vi "Begin.vi"() -> (0 "error out":errorcluster)   [LabVIEW 2013]
doc: "Called before other user functions, this VI is expected to open initial I/O refnums, load in file data, and do all program initialization. Notice that the <B>error out</B> terminal is simply used for data flow. Wiring it to other structures or subVIs ensures that this VI runs first."
uses:
  <vilib>/Rock Robotics/WPI/Joystick/WPI_JoystickDeviceEnum.ctl
  RefnameEnum.ctl
  RollerAction.ctl
  DoubleSolenoidAction.ctl
  CollectorAction.ctl
  <vilib>/Rock Robotics/SystemInterfaces/Typedef/FPGA_TypedefSolenoidModule.ctl
  <vilib>/Rock Robotics/WPI/Solenoid/WPI_SolenoidChannel.ctl
  <vilib>/Rock Robotics/SystemInterfaces/DIO/FPGA_DIOPWMChannel.ctl
  <vilib>/Rock Robotics/SystemInterfaces/Typedef/FPGA_TypedefDigitalModule.ctl
  <vilib>/Rock Robotics/SystemInterfaces/DIO/FPGA_DIOChannel.ctl
  <vilib>/Rock Robotics/SystemInterfaces/DIO/FPGA_DIORelayChannel.ctl
  <vilib>/Rock Robotics/WPI/Relay/WPI_RelayDirection.ctl
  <vilib>/Rock Robotics/WPI/Solenoid/WPI_SolenoidOpenSingle.vi
  <vilib>/Rock Robotics/WPI/MotorControl/WPI_MotorControlOpen Talon.vi
  <vilib>/Rock Robotics/WPI/Compressor/WPI_CompressorGetSetRefNum.vi
panel:
  # "SET AS DEFAULT"
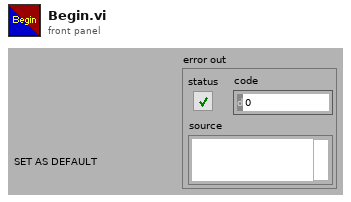
[diagram p1: front panel]
types:
  T1 = typedef "FPGA_DIOChannel.ctl" = enum8{"DIO 1", "DIO 2", "DIO 3", "DIO 4", "DIO 5", "DIO 6", "DIO 7", "DIO 8", "DIO 9", "DIO 10", "DIO 11", "DIO 12", "DIO 13", "DIO 14", "Invalid"}
  T2 = typedef "WPI_RelayDirection.ctl" = enum16{"Both directions", "Forward only", "Reverse only"}
  T3 = typedef "FPGA_DIORelayChannel.ctl" = enum8{"Relay 1", "Relay 2", "Relay 3", "Relay 4", "Relay 5", "Relay 6", "Relay 7", "Relay 8", "Invalid"}
  T4 = typedef "FPGA_TypedefDigitalModule.ctl" = enum16{"Digital Module 1", "Digital Module 2"}
  T5 = typedef "FPGA_DIOPWMChannel.ctl" = enum8{"PWM 1", "PWM 2", "PWM 3", "PWM 4", "PWM 5", "PWM 6", "PWM 7", "PWM 8", "PWM 9", "PWM 10", "Invalid"}
  T6 = typedef "WPI_SolenoidChannel.ctl" = enum8{"Solenoid 1", "Solenoid 2", "Solenoid 3", "Solenoid 4", "Solenoid 5", "Solenoid 6", "Solenoid 7", "Solenoid 8", "Invalid"}
  T7 = typedef "FPGA_TypedefSolenoidModule.ctl" = enum16{"Solenoid Module 1", "Solenoid Module 2"}
  T8 = typedef "CollectorAction.ctl" = enum16{"Init", "Raise", "Lower", "Stop", "GetStatus"}
  T9 = typedef "DoubleSolenoidAction.ctl" = enum16{"Init", "Middle", "In", "Out"}
  T10 = typedef "RefnameEnum.ctl" = enum16{"TankDrive", "Controller1", "Controller2", "SonicShifter", "Compressor"}
  T11 = typedef "RollerAction.ctl" = enum16{"Init", "Off", "Forward", "Reverse"}
  T12 = typedef "WPI_JoystickDeviceEnum.ctl" = enum16{"USB 1", "USB 2", "USB 3", "USB 4", "Kinect 1", "Kinect 2"}
  T13 = typedef "WPI_JoystickDevRef.ctl" = cluster{"Device":T12}
  T14 = typedef "WPI_MotorControlDeviceRef.ctl" = cluster{"DeviceStatus":errorcluster, "Type":enum16{"PWM", "CAN"}, "PWM":cluster{"Digital Module":T4, "PWM Channel":T5, "DeadBand":T15}, "CAN":cluster{"Device Number":u8, "Control Mode":T16, "Semaphore":T17, "Max Vout":dbl}, "Invert":bool, "TransformRef":T18, "InvTransformRef":T18}
  T15 = typedef "WPI_PWMDeadband.ctl" = cluster{"Name":string, "maxPositivePwm":i32, "minPositivePwm":i32, "centerPwm":i32, "maxNegativePwm":i32, "minNegativePwm":i32, "angularRange":u16}
  T16 = typedef "WPI_CANJaguar_ControlMode.ctl" = enum8{"Percent VBus", "Current", "Speed", "Position", "Voltage"}
  T17 = typedef "Semaphore RefNum" = refnum<k1>
  T18 = typedef "WPI_PWMTransform_ConPane.ctl" = refnum<vi>
  T19 = typedef "WPI_DigitalInputDevRef.ctl" = cluster{"DevStatus":errorcluster, "DIO Channel":T1, "Digital Module":T4}
  T20 = typedef "WPI_CompressorDevRef.ctl" = cluster{"DevStatus":errorcluster, "DigitalInputDevRef":T19, "RelayDevRef":T21}
  T21 = typedef "WPI_RelayDevRef.ctl" = cluster{"DevStatus":errorcluster, "Relay Channel":T3, "Digital Module":T4, "Relay Direction":T2}
  T22 = typedef "WPI_SolenoidDevRef.ctl" = cluster{"DevStatus":errorcluster, "Solenoid Module":T7, "Forward Solenoid Channel":T6, "Reverse Solenoid Channel":T6}
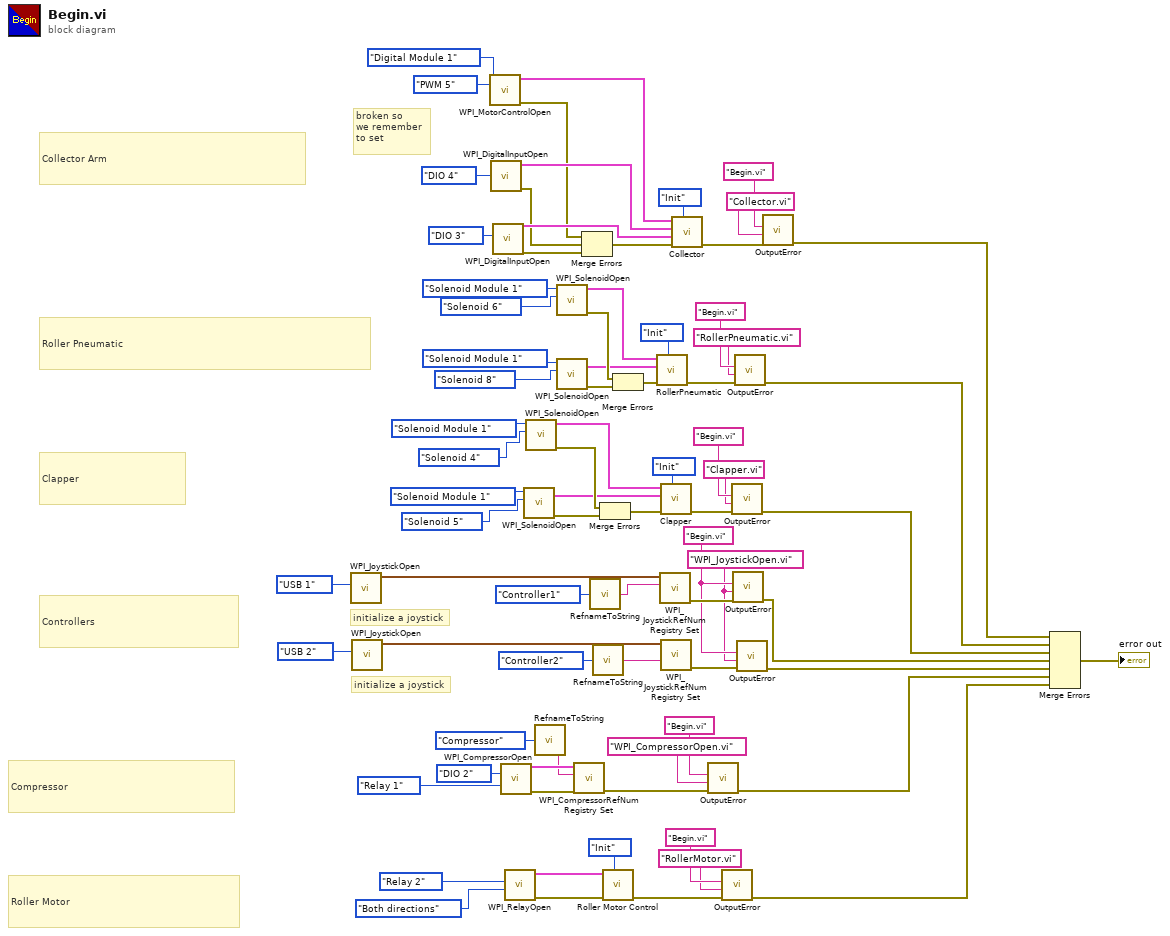
[diagram p0: block diagram]
diagram:
  w70 = "WPI_JoystickOpen.vi" ("Causing VI")
  w71 = "Begin.vi" ("Calling VI")
  # "broken so\nwe remember\nto set"
  # "Collector Arm"
  # "Roller Pneumatic"
  # "Clapper"
  # "Compressor"
  # "Roller Motor"
  # "Controllers"
  # "initialize a joystick"
  # "initialize a joystick"
  n1 = call <vilib>:"WPI_JoystickOpen.vi"("JoystickDevice"=WPI_JoystickDeviceEnum."USB 1") -> ("JoystickDevRef"=w77:T13)  [unwired: 10 in]
  n2 = call <vilib>:"WPI_JoystickOpen.vi"("JoystickDevice"=WPI_JoystickDeviceEnum."USB 2") -> ("JoystickDevRef"=w74:T13)  [unwired: 10 in]
  n3 = call-poly <vilib>:"WPI_MotorControlOpen.vi"("PWM Channel"=FPGA_DIOPWMChannel."PWM 5", "Digital Module (Module 1)"=FPGA_TypedefDigitalModule."Digital Module 1") -> ("error out"=w30:errorcluster, "MotorControlDeviceRef"=w36:T14)  [unwired: 8 in]
  n4 = call <vilib>:"WPI_DigitalInputOpen.vi"("DIO Channel"=FPGA_DIOChannel."DIO 4") -> ("error out"=w31:errorcluster, "DigitalInputDevRef"=w35:T19)  [unwired: 9 in]
  n5 = call <vilib>:"WPI_DigitalInputOpen.vi"("DIO Channel"=FPGA_DIOChannel."DIO 3") -> ("error out"=w32:errorcluster, "DigitalInputDevRef"=w34:T19)  [unwired: 9 in]
  n6 = call <vilib>:"WPI_CompressorOpen.vi"("Pressure Switch DIO Channel"=FPGA_DIOChannel."DIO 2", "Relay Channel"=FPGA_DIORelayChannel."Relay 1") -> ("CompressorDevRef"=w60:T20, "error out"=w59:errorcluster)  [unwired: 3 in, 9 out]
  n7 = call <vilib>:"WPI_RelayOpen.vi"("Relay Direction"=WPI_RelayDirection."Both directions", "Relay Channel"=FPGA_DIORelayChannel."Relay 2") -> ("error out"=w65:errorcluster, "RelayDevRef"=w63:T21)  [unwired: 8 in]
  n8 = call-poly <vilib>:"WPI_SolenoidOpen.vi"("Solenoid Channel"=WPI_SolenoidChannel."Solenoid 5", "Solenoid Module (Module 1)"=FPGA_TypedefSolenoidModule."Solenoid Module 1") -> ("error out"=w23:errorcluster, "SolenoidDevRef"=w22:T22)  [unwired: 8 in]
  n9 = call-poly <vilib>:"WPI_SolenoidOpen.vi"("Solenoid Channel"=WPI_SolenoidChannel."Solenoid 4", "Solenoid Module (Module 1)"=FPGA_TypedefSolenoidModule."Solenoid Module 1") -> ("error out"=w52:errorcluster, "SolenoidDevRef"=w51:T22)  [unwired: 8 in]
  n10 = call "RefnameToString.vi"("Enum"=RefnameEnum."Compressor") -> ("Refname"=w56:string)
  n11 = call-poly <vilib>:"WPI_SolenoidOpen.vi"("Solenoid Channel"=WPI_SolenoidChannel."Solenoid 6", "Solenoid Module (Module 1)"=FPGA_TypedefSolenoidModule."Solenoid Module 1") -> ("error out"=w42:errorcluster, "SolenoidDevRef"=w43:T22)  [unwired: 8 in]
  n12 = call-poly <vilib>:"WPI_SolenoidOpen.vi"("Solenoid Channel"=WPI_SolenoidChannel."Solenoid 8", "Solenoid Module (Module 1)"=FPGA_TypedefSolenoidModule."Solenoid Module 1") -> ("error out"=w18:errorcluster, "SolenoidDevRef"=w17:T22)  [unwired: 8 in]
  n13 = call <vilib>:"WPI_CompressorRefNum Registry Set.vi"("error in (no error)"=w59, "refnum name"=w56, "CompressorDevRef"=w60) -> ("error out"=w58:errorcluster)  [unwired: 7 in, 1 out]
  n14 = Merge Errors(w30, w31, w32) -> (w33:errorcluster)
  n15 = call "RefnameToString.vi"("Enum"=RefnameEnum."Controller1") -> ("Refname"=w68:string)
  n16 = call "RefnameToString.vi"("Enum"=RefnameEnum."Controller2") -> ("Refname"=w66:string)
  n17 = Merge Errors(w52, w23) -> (w24:errorcluster)
  n18 = call "Roller Motor Control.vi"("Action"=RollerAction."Init" ("RollerState"), "Error in"=w65, "RelayDevRef"=w63) -> ("Error out"=w64:errorcluster)  [unwired: 8 in]
  n19 = Merge Errors(w42, w18) -> (w19:errorcluster)
  n20 = call "RollerPneumatic.vi"("State"=DoubleSolenoidAction."Init", "Error in"=w19, "Plugged"=w17, "Open"=w43) -> ("Error out"=w46:errorcluster)  [unwired: 7 in]
  n21 = call <vilib>:"WPI_JoystickRefNum Registry Set.vi"("refnum name"=w68, "JoystickDevRef"=w77) -> ("error out"=w72:errorcluster)  [unwired: 8 in, 1 out]
  n22 = call "Clapper.vi"("State"=DoubleSolenoidAction."Init", "Error in"=w24, "Plugged"=w22, "Open"=w51) -> ("Error out"=w50:errorcluster)  [unwired: 7 in]
  n23 = call <vilib>:"WPI_JoystickRefNum Registry Set.vi"("refnum name"=w66, "JoystickDevRef"=w74) -> ("error out"=w73:errorcluster)  [unwired: 8 in, 1 out]
  n24 = call "Collector.vi"("Action"=CollectorAction."Init", "Error in"=w33, "BottomLS"=w34, "TopLS"=w35, "Motor"=w36) -> ("Error out"=w38:errorcluster)  [unwired: 4 in, 2 out]
  n25 = call "OutputError.vi"("error in (no error)"=w58, "Causing VI"="WPI_CompressorOpen.vi", "Calling VI"="Begin.vi") -> ("error out"=w2:errorcluster)  [unwired: 8 in]
  n26 = call "OutputError.vi"("error in (no error)"=w64, "Causing VI"="RollerMotor.vi", "Calling VI"="Begin.vi") -> ("error out"=w1:errorcluster)  [unwired: 8 in]
  n27 = call "OutputError.vi"("error in (no error)"=w50, "Causing VI"="Clapper.vi", "Calling VI"="Begin.vi") -> ("error out"=w27:errorcluster)  [unwired: 8 in]
  n28 = call "OutputError.vi"("error in (no error)"=w72, "Causing VI"=w70, "Calling VI"=w71) -> ("error out"=w26:errorcluster)  [unwired: 8 in]
  n29 = call "OutputError.vi"("error in (no error)"=w46, "Causing VI"="RollerPneumatic.vi", "Calling VI"="Begin.vi") -> ("error out"=w28:errorcluster)  [unwired: 8 in]
  n30 = call "OutputError.vi"("error in (no error)"=w73, "Causing VI"=w70, "Calling VI"=w71) -> ("error out"=w25:errorcluster)  [unwired: 8 in]
  n31 = call "OutputError.vi"("error in (no error)"=w38, "Causing VI"="Collector.vi", "Calling VI"="Begin.vi") -> ("error out"=w29:errorcluster)  [unwired: 8 in]
  n32 = Merge Errors(w29, w28, w27, w26, w25, w2, w1) -> (→"error out":errorcluster)
